vi "Push_Data_via_Public_Client.vi"(5 "Archive File?":bool[](array[boolean]), 6 "application reference":refnum<vi>, 7 "error in (no error)":errorcluster, 8 "Running on Server?":bool, 10 "Path of Files relative to EnFlo Data Root":path[](array[path])) -> (0 "error out":errorcluster, 2 "Problem Files":path[](array[path]), 3 "Error String":string)   [LabVIEW 2018]
uses:
  Anemometry/Anemometry Sub Vis/Globals/Constants_global.vi
  Sub VIs/Harvest_Global.vi
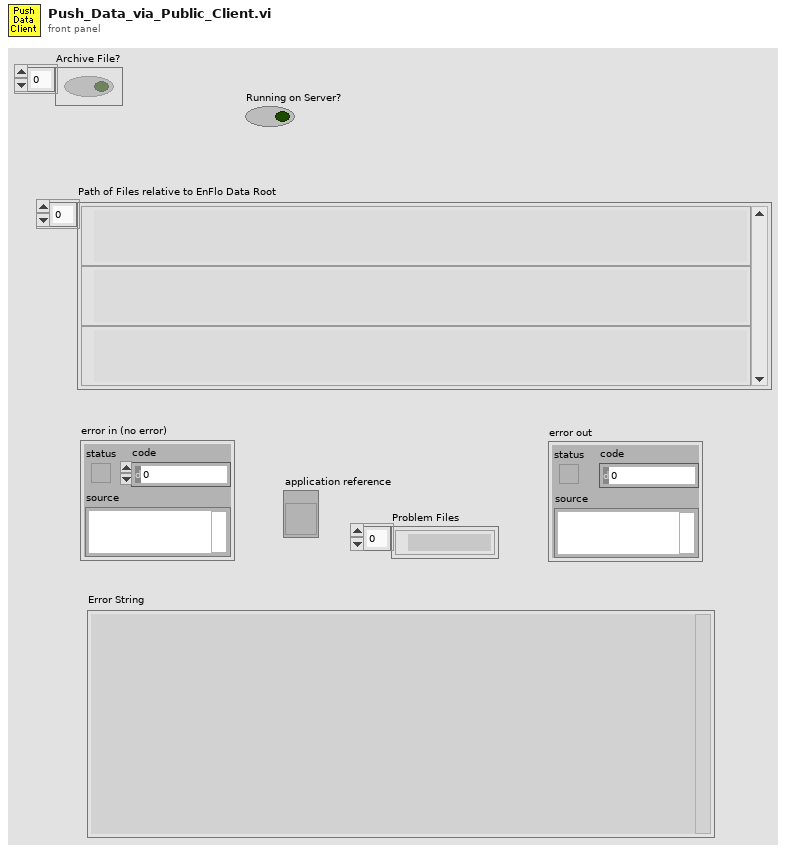
[diagram p1: front panel]
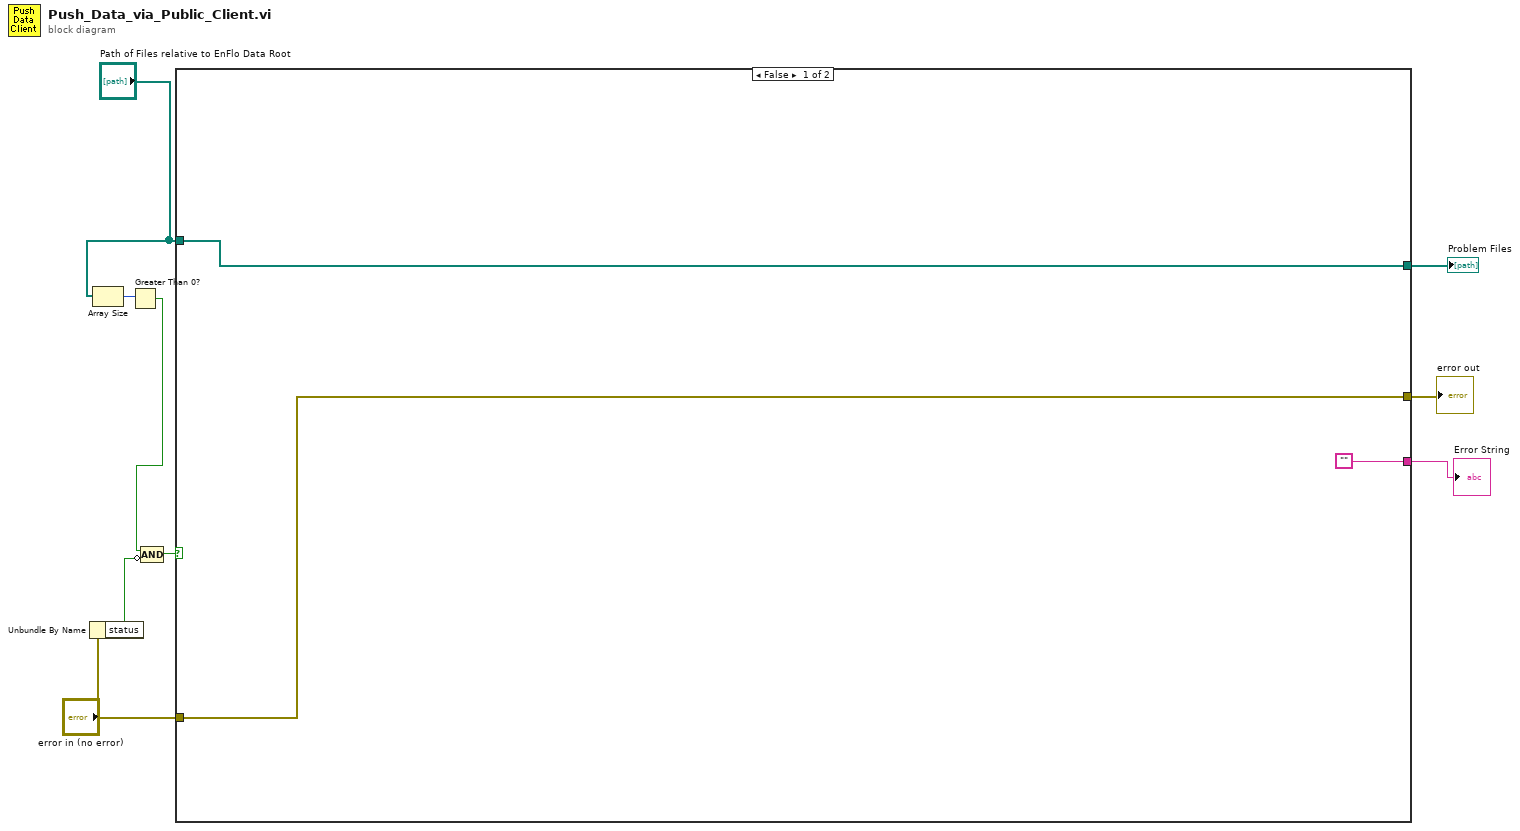
[diagram p0: block diagram]
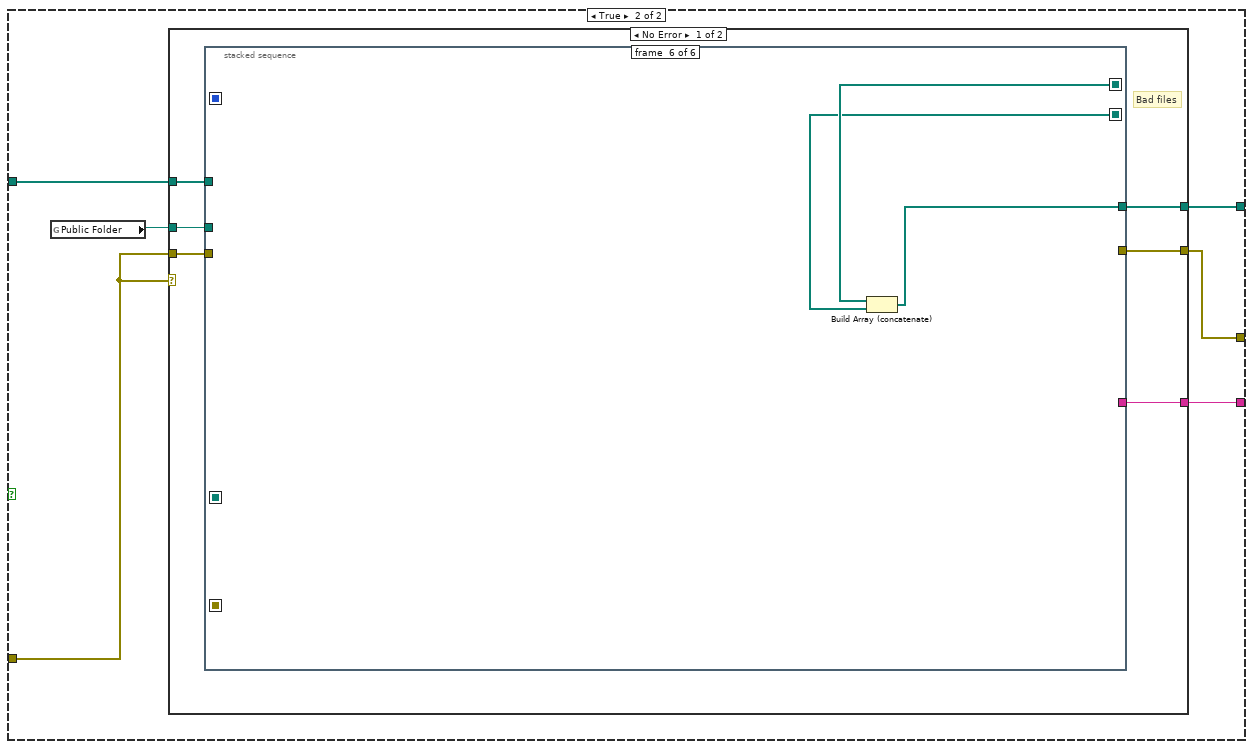
[diagram p2: hidden frame]
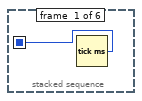
[diagram p3: hidden frame]
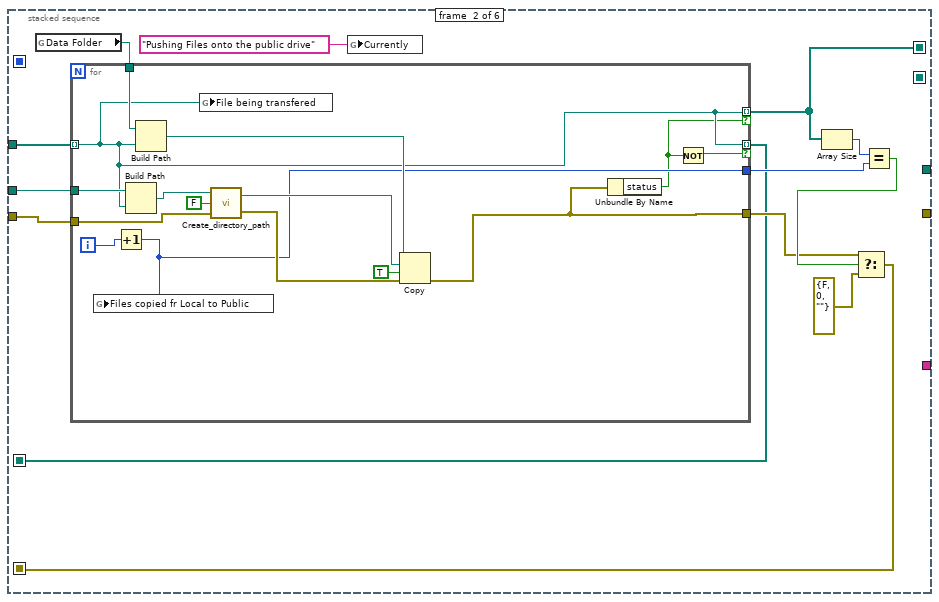
[diagram p4: hidden frame]
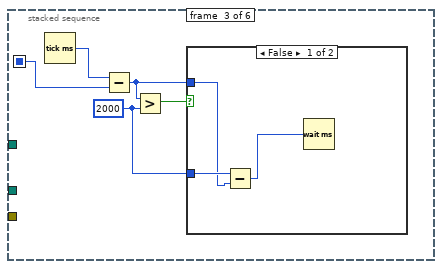
[diagram p5: hidden frame]
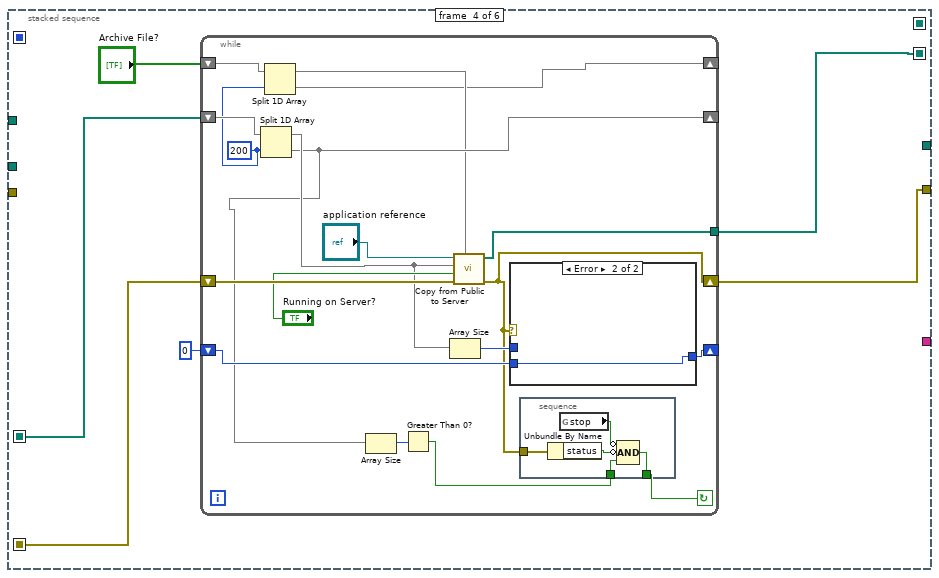
[diagram p7: hidden frame]
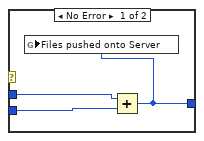
[diagram p8: hidden frame]
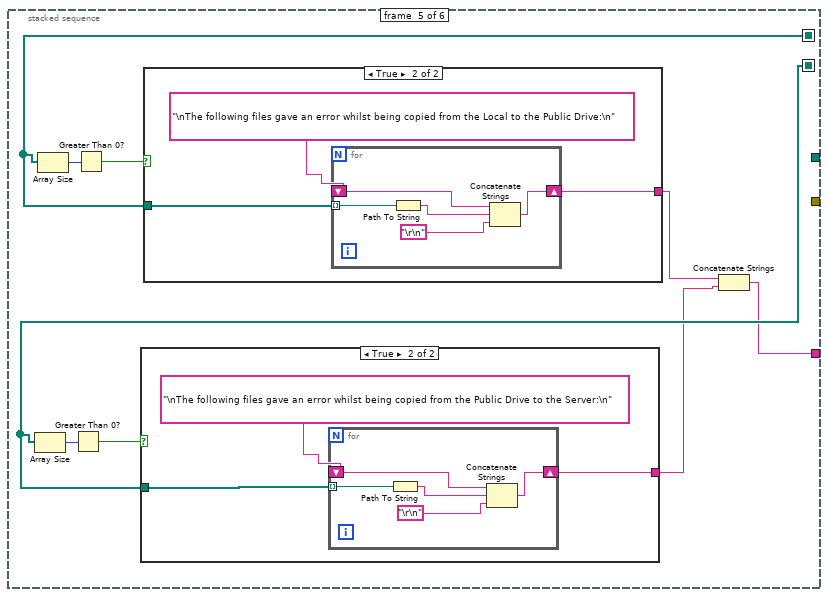
[diagram p9: hidden frame]
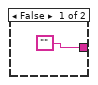
[diagram p10: hidden frame]
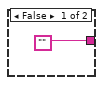
[diagram p11: hidden frame]
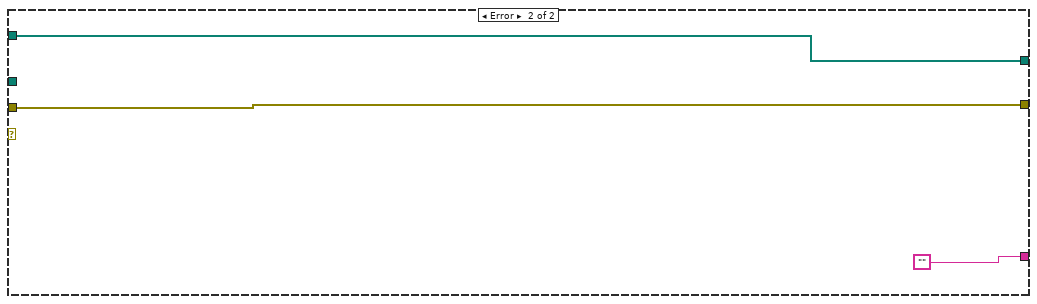
[diagram p12: hidden frame]
diagram:
  n1 = Unbundle By Name("error in (no error)") -> ("status"=w4:bool)
  n2 = Array Size(array="Path of Files relative to EnFlo Data Root") -> (size(s)=w7:i32)
  n3 = Greater Than 0?(x=w7) -> (x > 0?=w5:bool)
  n4 = Compound Arithmetic op=AND(w5, invert w4) -> (w3:bool)
  n5 = case shown="False" w3 {
    tunnel: [w12 w15] -> w9
    tunnel: "error in (no error)" -> [w12 w18]
    tunnel: "Path of Files relative to EnFlo Data Root" -> [w10 w16]
    tunnel: ["" w14] -> w2
    tunnel: [w10 w13] -> w1
    frame False {
    }
    frame True {
      n6 = global read "Constants_global.vi" "Public Folder"() -> (w17:path)
      n7 = case shown="No Error" w18 {
        tunnel: [w21 w127] -> w15
        tunnel: w18 -> [w22 w127]
        tunnel: w16 -> [w24 w125]
        tunnel: w17 -> [w23 _]
        tunnel: [w20 ""] -> w14
        tunnel: [w19 w125] -> w13
        frame No Error {
          # "Bad files"
          n8 = stacked-sequence {
            seq-local: [w25 _ _ _ _ _] -> [_ _ w57 _ _ _]
            seq-local: [_ w28 _ _ _ _] -> [_ _ _ w67 _ _]
            seq-local: [_ w27 _ _ _ _] -> [_ _ _ _ w103 w124]
            seq-local: [_ w26 _ _ _ _] -> [_ _ _ w63 _ _]
            seq-local: [_ _ _ w62 _ _] -> [_ _ _ _ w98 w123]
            tunnel: w24 -> [_ w37 _ _ _ _]
            tunnel: w23 -> [_ w36 _ _ _ _]
            tunnel: w22 -> [_ w35 _ _ _ _]
            tunnel: [_ _ _ w66 _ _] -> w21
            tunnel: [_ _ _ _ w95 _] -> w20
            tunnel: [_ _ _ _ _ w122] -> w19
            frame #0 {
              n9 = Tick Count (ms)() -> (millisecond timer value=w25:u32)
            }
            frame #1 {
              n10 = global read "Constants_global.vi" "Data Folder"() -> (w38:path)
              n11 = for {
                tunnel: w38 -> [w47]
                tunnel: w37 -> [w41] mode=indexing
                tunnel: w36 -> [w51]
                tunnel: w35 -> [w48]
                tunnel: [w44] -> w29
                tunnel: [w41] -> w27 mode=indexing if=w40
                tunnel: [w43] -> w32
                tunnel: [w41] -> w26 mode=indexing if=w39
                i -> [w46]
                n12 = Increment(x=w46) -> (x+1=w43:i32)
                n13 = global write "Harvest_Global.vi" "Files copied fr Local to Public"(w43) -> ()
                n14 = Build Path(base path=w51, name or relative path=w41) -> (appended path=w52:path)
                n15 = Build Path(base path=w47, name or relative path=w41) -> (appended path=w53:path)
                n16 = global write "Harvest_Global.vi" "File being transfered"(w41) -> ()
                n17 = call "Create_directory_path.vi"("error in (no error)"=w48, "Dialog Box"=FALSE, "Path name"=w52) -> ("error out"=w49:errorcluster, "Path name Out"=w50:path)
                n18 = Copy(8:w49, 9:TRUE ("overwrite (F)"), 10:w50, 11:w53) -> (0:w44:errorcluster)  [unwired: 1 in, 2 out]
                n19 = Unbundle By Name(w44) -> ("status"=w40:bool)
                n20 = Not(x=w40) -> (.not. x?=w39:bool)
              }
              n21 = global write "Harvest_Global.vi" "Currently"("Pushing Files onto the public drive" ("Currently Running")) -> ()
              n22 = Array Size(array=w27) -> (size(s)=w33:i32)
              n23 = Equal?(x=w33, y=w32) -> (x = y?=w30:bool)
              n24 = Select(t=w29, s=w30, f=errorcluster {"status"=FALSE, "code"=0, "source"=""} ("error out")) -> (s? t:f=w28:errorcluster)
            }
            frame #2 {
              w55 = u32 2000 ("y")
              n25 = Tick Count (ms)() -> (millisecond timer value=w58:u32)
              n26 = Subtract(x=w58, y=w57) -> (x-y=w54:u32)
              n27 = Greater?(x=w54, y=w55) -> (0:w56:bool)
              n28 = case shown="False" w56 {
                tunnel: w55 -> [w61 _]
                tunnel: w54 -> [w60 _]
                frame False {
                  n29 = Subtract(x=w61, y=w60) -> (x-y=w59:u32)
                  n30 = Wait (ms)(milliseconds to wait=w59) -> ()  [unwired: 1 out]
                }
                frame True {
                }
              }
            }
            frame #3 {
              n31 = while {
                shift-right: [w77] -> w66
                shift-left: w67 -> [w85]
                shift-right: [w76] -> _
                shift-left: w63 -> [w82]
                shift-right: [w79] -> _
                shift-left: 0 -> [w78]
                shift-right: [w69] -> _
                shift-left: "Archive File?" -> [w72]
                tunnel: [w68] -> w62
                stop <- w73 continue-if-true
                w71 = 200 ("index")
                n32 = Split 1D Array(array=w82, index=w71) -> (first subarray=w81:path[], second subarray=w76:path[])
                n33 = Split 1D Array(array=w72, index=w71) -> (first subarray=w70:bool[], second subarray=w69:bool[])
                n34 = Array Size(array=w76) -> (size(s)=w75:i32)
                n35 = Greater Than 0?(x=w75) -> (x > 0?=w74:bool)
                n36 = Array Size(array=w81) -> (size(s)=w80:i32)
                n37 = call "Copy from Public to Server.vi"("Archive File?"=w70, "error in (no error)"=w85, "Running on Server?"="Running on Server?", "Path of Files relative to EnFlo Data Root"=w81, "Application in"="application reference") -> ("error out"=w77:errorcluster, "Problem Files"=w68:path[])  [unwired: 5 in]
                n38 = case shown="Error" w77 {
                  tunnel: w80 -> [w93 _]
                  tunnel: [w91 w94] -> w79
                  tunnel: w78 -> [w92 w94]
                  frame No Error {
                    n39 = Add(x=w93, y=w92) -> (x+y=w91:i32)
                    n40 = global write "Harvest_Global.vi" "Files pushed onto Server"(w91) -> ()
                  }
                  frame Error {
                  }
                }
                n41 = stacked-sequence {
                  tunnel: [w89] -> w73
                  tunnel: w77 -> [w87]
                  tunnel: w74 -> [w86]
                  frame #0 {
                    n42 = Unbundle By Name(w87) -> ("status"=w90:bool)
                    n43 = global read "Harvest_Global.vi" "stop"() -> (w88:bool)
                    n44 = Compound Arithmetic op=AND(invert w88, invert w90, w86) -> (w89:bool)
                  }
                }
              }
            }
            frame #4 {
              n45 = Array Size(array=w98) -> (size(s)=w99:i32)
              n46 = Array Size(array=w103) -> (size(s)=w102:i32)
              n47 = Greater Than 0?(x=w99) -> (x > 0?=w100:bool)
              n48 = Greater Than 0?(x=w102) -> (x > 0?=w101:bool)
              n49 = case shown="True" w100 {
                tunnel: w98 -> [_ w107]
                tunnel: ["" w105] -> w96
                frame False {
                }
                frame True {
                  n50 = for {
                    tunnel: w107 -> [w112] mode=indexing
                    shift-right: [w109] -> w105
                    shift-left: "\nThe following files gave an error whilst being copied from the Public Drive to the Server:\n" -> [w108]
                    n51 = Path To String(path=w112) -> (string=w111:string)
                    n52 = Concatenate Strings(w108, w111, "\r\n") -> (w109:string)
                  }
                }
              }
              n53 = case shown="True" w101 {
                tunnel: w103 -> [_ w116]
                tunnel: ["" w114] -> w97
                frame False {
                }
                frame True {
                  n54 = for {
                    tunnel: w116 -> [w121] mode=indexing
                    shift-right: [w118] -> w114
                    shift-left: "\nThe following files gave an error whilst being copied from the Local to the Public Drive:\n" -> [w117]
                    n55 = Path To String(path=w121) -> (string=w120:string)
                    n56 = Concatenate Strings(w117, w120, "\r\n") -> (w118:string)
                  }
                }
              }
              n57 = Concatenate Strings(w97, w96) -> (w95:string)
            }
            frame #5 {
              n58 = Build Array (concatenate)(w124, w123) -> (w122:path[])
            }
          }
        }
        frame Error {
        }
      }
    }
  }
  "error out" <- w9
  "Error String" <- w2
  "Problem Files" <- w1
